vi "Settings Dialog.vi"(8 "error in (no error)":cluster{"状态":bool, "代码":i32, "源":string} caption="错误输入（无错误）", 11 "设置输入":T1) -> (0 "error out":cluster{"状态":bool, "代码":i32, "源":string} caption="错误输出", 1 "取消？":bool, 2 "需要刷新UI？":bool, 3 "设置输出":T1)   [LabVIEW 2012, in "Settings.lvlib"]
doc: "用于选择用户设置的对话框。"
uses:
  Settings.lvlib
  Settings.ctl
  Acquisition/Hardware Configuration.ctl
  Acquisition/Signal Type.ctl
  Logging/Logging Configuration.ctl
  <vilib>/Instr/_visa.llb/VISA Configure Serial Port (Instr).vi
  <vilib>/Utility/xml.llb/Write to XML File(string).vi
  Acquisition/Acquisition.lvlib
  Logging/Logging.lvlib
panel:
  in  "硬件配置.VISA资源名称":refnum<visa-resource-name>
  in  "记录文件路径":path
  in  "信号类型":u16(ring) items=["正弦波", "方波（带噪声）"]
  in  "取消按钮":bool
  in  "确定按钮":bool
  # "对话框不可见部分（用于连线板）"
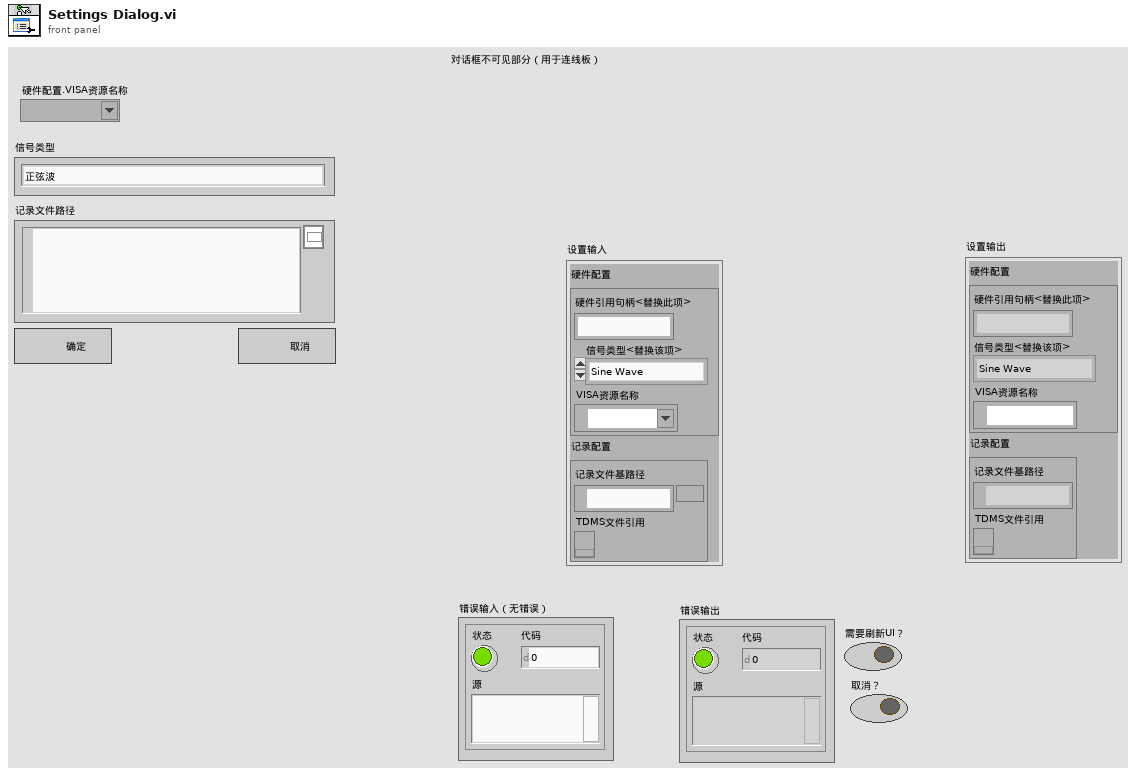
[diagram p1: front panel]
types:
  T1 = typedef "Settings.lvlib/Settings.ctl" = cluster{"硬件配置":T2, "记录配置":T4}
  T2 = typedef "Acquisition.lvlib/Hardware Configuration.ctl" = cluster{"硬件引用句柄<替换此项>":string, "信号类型<替换该项>":T3, "VISA资源名称":refnum<visa-resource-name>}
  T3 = typedef "Acquisition.lvlib/Signal Type.ctl" = enum16{"Sine Wave", "Square with Noise"}
  T4 = typedef "Logging.lvlib/Logging Configuration.ctl" = cluster{"记录文件基路径":path, "TDMS文件引用":refnum<k34>}
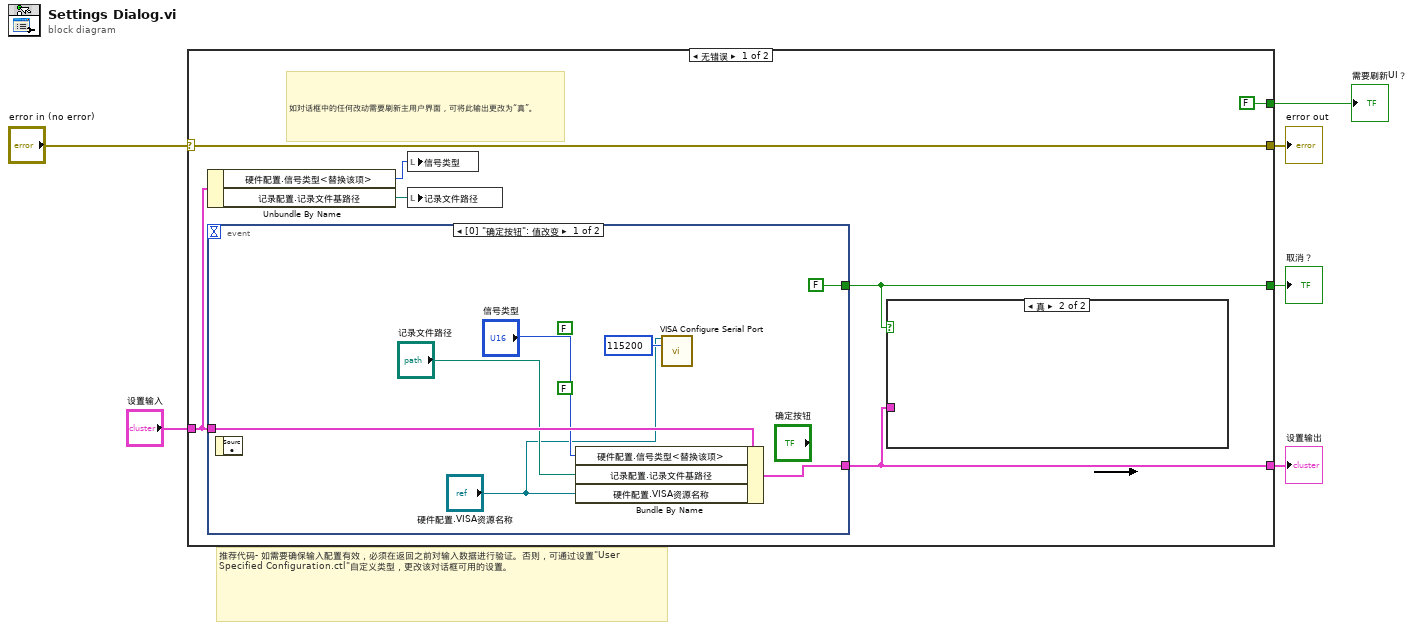
[diagram p0: block diagram]
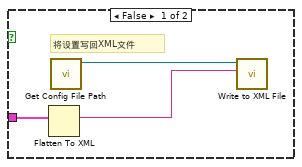
[diagram p2: hidden frame]
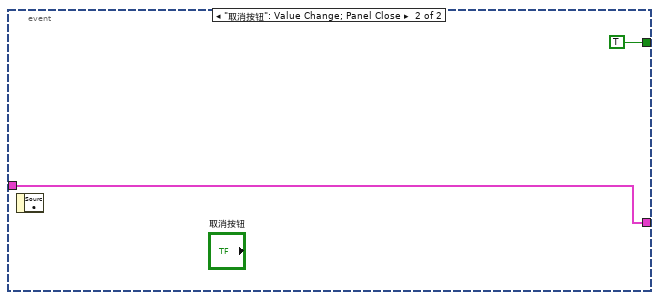
[diagram p3: hidden frame]
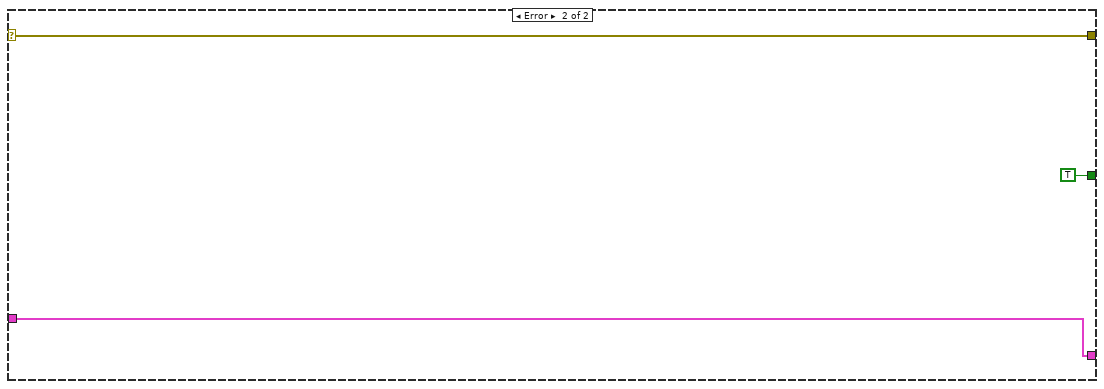
[diagram p4: hidden frame]
diagram:
  # "推荐代码- 如需要确保输入配置有效，必须在返回之前对输入数据进行验证。否则，可通过设置\"User Specified Configuration.ctl\"自定义类型，更改该对话框可用的设置。"
  n1 = case shown="无错误" "error in (no error)" {
    selector: "error in (no error)" -> [w13 w28]
    tunnel: [w13 w28] -> w5
    tunnel: "设置输入" -> [w9 w27]
    tunnel: [w10 w27] -> w3
    tunnel: [FALSE ("UI Refresh Needed?") _] -> w2
    tunnel: [w11 TRUE ("UI Refresh Needed?")] -> w1
    frame No Error {
      # "如对话框中的任何改动需要刷新主用户界面，可将此输出更改为“真”。"
      n2 = Unbundle By Name(w9) -> ("硬件配置.信号类型<替换该项>"=w8:T3, "记录配置.记录文件基路径"=w7:path)
      n3 = event shown="[0] \"确定按钮\": 值改变" {
        selector: _ -> [_ _]
        dyn-events: _ -> [_ _]
        timeout: _ -> [_ _]
        tunnel: [w21 w25] -> w10
        tunnel: w9 -> [w22 w25]
        tunnel: [FALSE ("UI Refresh Needed?") TRUE ("UI Refresh Needed?")] -> w11
        event "确定按钮": Value Change {
          (unwired) FALSE ("左后退按钮")
          (unwired) FALSE ("左前进按钮")
          n4 = event-data() -> ()  [unwired: 1 in, 1 out]
          n5 = Bundle By Name(cluster=w22, "硬件配置.信号类型<替换该项>"="信号类型", "记录配置.记录文件基路径"="记录文件路径", "硬件配置.VISA资源名称"="硬件配置.VISA资源名称") -> (w21:T1)
          n6 = call-poly "VISA Configure Serial Port"("VISA resource name"="硬件配置.VISA资源名称", "baud rate (9600)"=u32 115200) -> ()  [unwired: 12 in, 2 out]
        }
        event "取消按钮": Value Change; Panel Close {
          n7 = event-data() -> ()  [unwired: 1 in, 1 out]
        }
      }
      n8 = local write "信号类型"(w8) -> ()
      n9 = local write "记录文件路径"(w7) -> ()
      n10 = case shown="真" w11 {
        tunnel: w10 -> [w15 _]
        frame False {
          # "将设置写回XML文件"
          n11 = Flatten To XML(anything=w15) -> (xml string=w14:string)
          n12 = call "Get Config File Path.vi"() -> ("XML文件路径"=w16:path)  [unwired: 10 in, 1 out]
          n13 = call-poly <vilib>:"Write to XML File.vi"("XML Input"=w14, "XML File Path"=w16) -> ()  [unwired: 7 in, 3 out]
        }
        frame True {
        }
      }
    }
    frame Error {
    }
  }
  "需要刷新UI？" <- w2
  "error out" <- w5
  "设置输出" <- w3
  "取消？" <- w1
